vi "Zadanie2ArturCiapala.vi"() -> ()   [LabVIEW 2021]
panel:
  in  "N ostatnich pomiarów":i32=10
  out "T min":dbl
  out "T max":dbl
  in  "Próg dolny":dbl(knob) scale=0.0..50.0 scale format="%#_4g"
  in  "Próg górny":dbl(knob)=20.0 scale=0.0..50.0 scale format="%#_4g"
  in  "Zapis do pliku":bool
  out "Alarm dolny":bool
  out "Alarm górny":bool
  out "T chwilowe":dbl format="%#_4g"
  out "T usrednione":dbl format="%#_4g"
  in  "stop":bool
  out "Temperatura":T1(graph)
  in  "Adres zapisu pliku":path=path "C:/Users/userl/Desktop/Arturro/dane.txt"
  in  "Adres URL":string="dstp://10.42.14.223/temperatura"
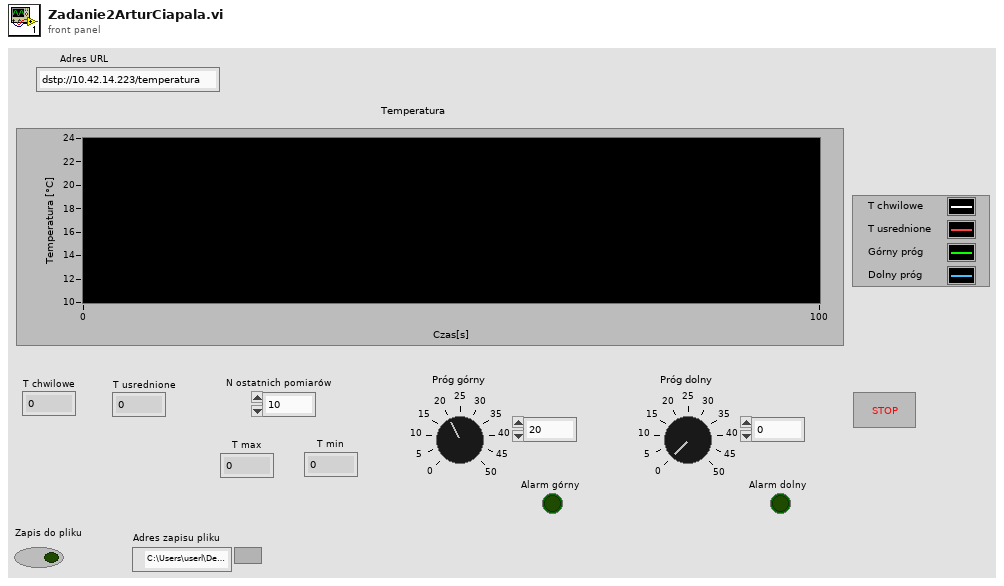
[diagram p1: front panel]
types:
  T1 = cluster{dbl, dbl, "Próg Górny":dbl, "Próg Dolny":dbl}
  T2 = enum16{"Read", "Write", "ReadWrite", "BufferedRead", "BufferedReadWrite"}
  T3 = enum16{"open", "replace", "create", "open or create", "replace or create", "replace or create with confirmation"}
  T4 = cluster{dbl, dbl, "Próg górny":dbl, "Próg dolny":dbl}
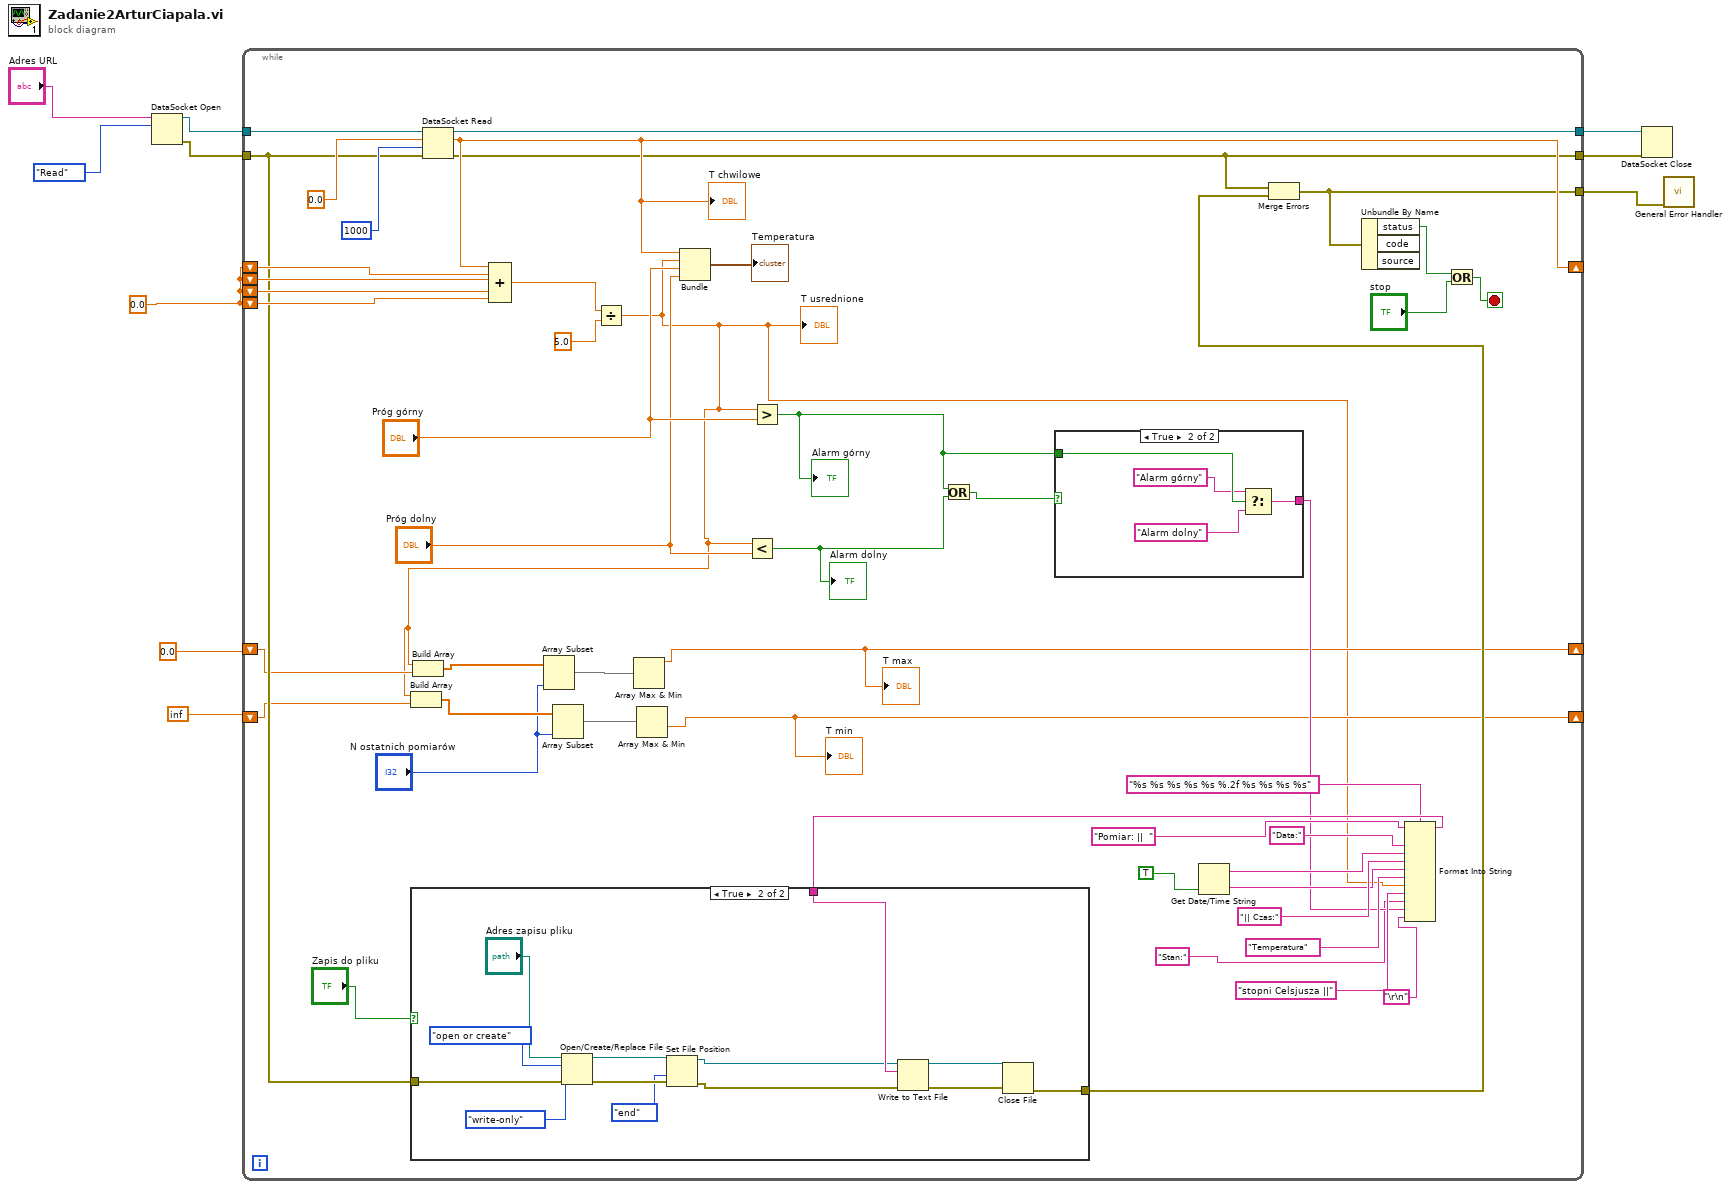
[diagram p0: block diagram]
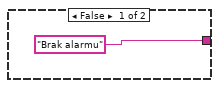
[diagram p2: hidden frame]
diagram:
  w5 = 0.0
  n1 = DataSocket Open(10:T2."Read" ("mode"), 11:"Adres URL") -> (0:w7:errorcluster, 3:w9:refnum<k13>)  [unwired: 2 in]
  n2 = while {
    shift-right: [w44] -> _
    shift-left: w5 -> [w56]
    shift-left: w5 -> [w55]
    shift-left: w5 -> [w54]
    shift-left: w5 -> [w53]
    tunnel: w9 -> [w58]
    tunnel: [w57] -> w8
    tunnel: w7 -> [w31]
    tunnel: [w29] -> w6
    tunnel: [w28] -> w4
    shift-right: [w17] -> _
    shift-left: 0.0 -> [w20]
    shift-right: [w16] -> _
    shift-left: inf -> [w14]
    stop <- w46 stop-if-true
    n3 = DataSocket Read(8:w31, 9:1000, 10:0.0, 11:w58) -> (0:w29:errorcluster, 2:w44:dbl, 3:w57:refnum<k13>)  [unwired: 1 in, 4 out]
    "T chwilowe" <- w44
    n4 = Compound Arithmetic op=ADD(w44, w56, w55, w54, w53) -> (w51:dbl)
    n5 = Divide(x=w51, y=5.0) -> (x/y=w15:dbl)
    "T usrednione" <- w15
    n6 = Build Array(w15, w14) -> (w13:dbl[])
    n7 = Build Array(w15, w20) -> (w19:dbl[])
    n8 = Array Subset(array=w19, length="N ostatnich pomiarów") -> (w18:dbl[])  [unwired: 1 in]
    n9 = Array Subset(array=w13, length="N ostatnich pomiarów") -> (w11:dbl[])  [unwired: 1 in]
    n10 = Array Max & Min(array=w18) -> (max value=w17:dbl)  [unwired: 3 out]
    "T max" <- w17
    n11 = Array Max & Min(array=w11) -> (min value=w16:dbl)  [unwired: 3 out]
    "T min" <- w16
    n12 = Bundle(w44, w15, "Próg górny"="Próg górny", "Próg dolny"="Próg dolny") -> (→"Temperatura":T4)  [unwired: 1 in]
    n13 = Less?(x=w15, y="Próg dolny") -> (x < y?=w43:bool)
    "Alarm dolny" <- w43
    n14 = Greater?(x=w15, y="Próg górny") -> (0:w41:bool)
    "Alarm górny" <- w41
    n15 = Or(x=w41, y=w43) -> (x .or. y?=w42:bool)
    n16 = case shown="True" w42 {
      tunnel: w41 -> [_ w63]
      tunnel: ["Brak alarmu" w60] -> w22
      frame False {
      }
      frame True {
        n17 = Select(t="Alarm górny", s=w63, f="Alarm dolny") -> (s? t:f=w60:string)
      }
    }
    n18 = Get Date/Time String(want seconds? (F)=TRUE) -> (date string=w38:string, time string=w36:string)  [unwired: 2 in]
    n19 = Format Into String(format string="%s %s %s %s %s %.2f %s %s %s %s", initial string="Pomiar: ||  ", "Data:", w38, "|| Czas:", w36, "Temperatura", w15, "stopni Celsjusza ||", "Stan:", w22, "\r\n") -> (resulting string=w33:string)  [unwired: 1 in, 1 out]
    n20 = case shown="True" "Zapis do pliku" {
      tunnel: w33 -> [_ w77]
      tunnel: w31 -> [w64 w73]
      tunnel: [w64 w72] -> w30
      frame False {
      }
      frame True {
        n21 = Open/Create/Replace File(file path (use dialog)="Adres zapisu pliku", error in=w73, operation (0:open)=T3."open or create", access (0:read/write)=enum16{"read/write", "read-only", "write-only"}."write-only") -> (refnum out=w70:refnum<file>, error out=w76:errorcluster)  [unwired: 2 in, 1 out]
        n22 = Set File Position(refnum=w70, from (0:start)=enum16{"start", "end", "current"}."end", error in=w76) -> (refnum out=w69:refnum<file>, error out=w75:errorcluster)  [unwired: 1 in]
        n23 = Write to Text File(file (use dialog)=w69, text=w77, error in=w75) -> (refnum out=w68:refnum<file>, error out=w74:errorcluster)  [unwired: 1 in, 1 out]
        n24 = Close File(refnum=w68, error in=w74) -> (error out=w72:errorcluster)  [unwired: 1 out]
      }
    }
    n25 = Merge Errors(w29, w30) -> (w28:errorcluster)
    n26 = Unbundle By Name(w28) -> ("status"=w48:bool)  [unwired: 2 out]
    n27 = Or(x=w48, y="stop") -> (x .or. y?=w46:bool)
  }
  n28 = DataSocket Close(8:w6, 11:w8) -> ()  [unwired: 1 in, 2 out]
  n29 = call <vilib>:"General Error Handler.vi"("error in (no error)"=w4) -> ()  [unwired: 10 in, 5 out]
